vi "Saturation Save Data.vi"(0 "TraceData":dbl[][](array[numeric]), 5 "start path":path=path "", 7 "Filename Note":string, 9 "Position":dbl[](array[numeric]), 11 "error in (no error)":errorcluster) -> (15 "error out":errorcluster)   [LabVIEW 2023]
uses:
  <vilib>/Utility/file.llb/Write Delimited Spreadsheet (DBL).vi
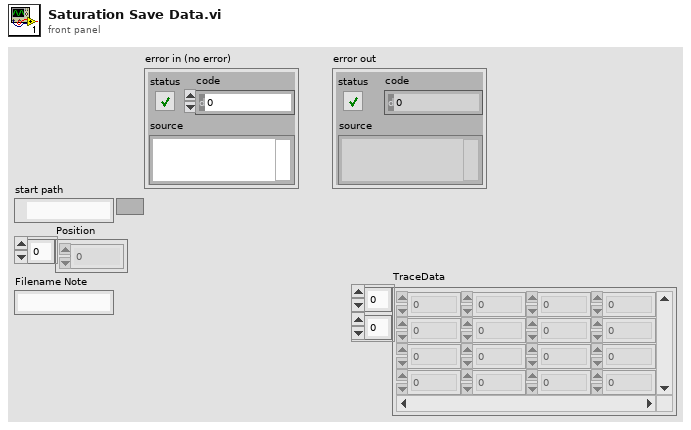
[diagram p1: front panel]
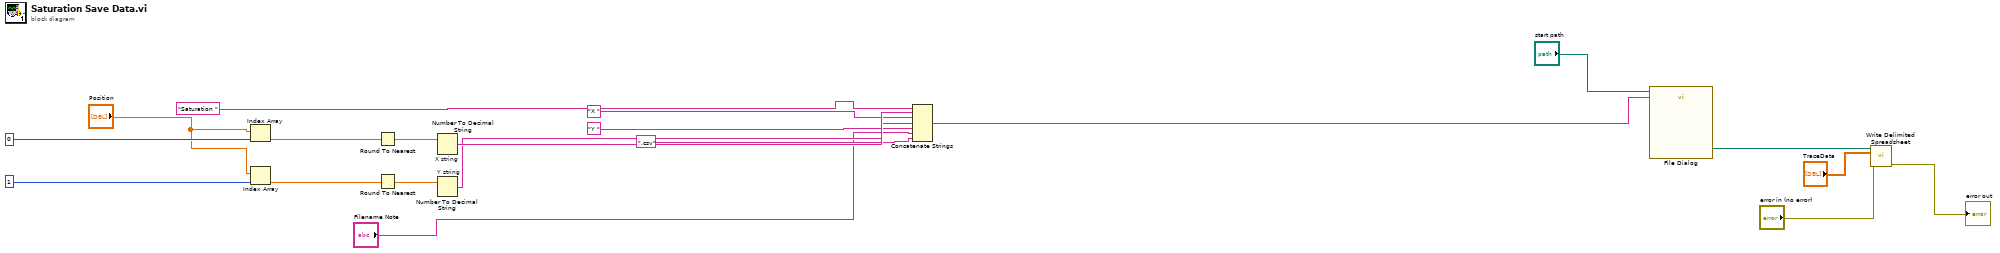
[diagram p0: block diagram]
diagram:
  n1 = Index Array(array="Position", index=0) -> (element=w18:dbl)
  n2 = Index Array(array="Position", index=1) -> (element=w17:dbl)
  n3 = Round To Nearest(number=w18) -> (nearest integer value=w19:dbl)
  n4 = Round To Nearest(number=w17) -> (nearest integer value=w20:dbl)
  n5 = Number To Decimal String "X string"(number=w19) -> (decimal integer string=w11:string)  [unwired: 1 in]
  n6 = Number To Decimal String "Y string"(number=w20) -> (decimal integer string=w9:string)  [unwired: 1 in]
  n7 = Concatenate Strings("Saturation ", w11, "X ", w9, "Y ", "Filename Note", ".csv") -> (w14:string)
  n8 = call "File Dialog"("start path"="start path", "default name"=w14) -> ("selected path"=w13:path)  [unwired: 10 in, 3 out]
  n9 = call-poly <vilib>:"Write Delimited Spreadsheet.vi"("file path (dialog if empty)"=w13, "2D data"="TraceData", "error in (no error)"="error in (no error)") -> ("error out"=→"error out":errorcluster)  [unwired: 11 in, 1 out]
